vi "Partridge.vi"() -> ()   [LabVIEW 2012]
uses:
  <vilib>/picture/picture.llb/imagedata.ctl
  <vilib>/xml/Load XML String.vi
  <vilib>/xml/NI_XML.lvlib
  <resource>/objmgr/DOMUserDefRef.rc
panel:
  in  "XML Menu":string="<?xml version=\"1.0\" encoding=\"ISO-8859-1\"?>\n<Menu>\n<Starters>\n<Starter>\n<Name>Soup</Name>\n<Desc>A hearty winter vegetable soup.</Desc>\n</Starter>\n<Starter>\n<Name>Salmon</Name>\n<Desc>Scottish smoked salmon.</Desc>\n</Starter>\n</Starters>\n<Mains>\n<Main>\n<Name>Roast Turkey</Name>\n<Desc>With all the trimmings!</Desc>\n</Main>\n<Main>\n<Name>Fillet of Sea Bass</Name>\n<Desc>With lemon and thyme fondant.</Desc>\n</Main>\n<Main>\n<Name>Shepherd's Pie</Name>\n<Desc>With Puy lentils and vegetables.</Desc>\n</Main>\n</Mains>\n<Desserts>\n<Dessert>\n<Name>Christmas Pudding</Name>\n<Desc>The traditional favourite.</Desc>\n</Dessert>\n<Dessert>\n<Name>Rich Chocolate Tart</Name>\n<Desc>With orage chantilly creme.</Desc>\n</Dessert>\n</Desserts>\n</Menu>"
  in  "Christmas Tree View":string(tree)
  # "A Partridge in a Pear Tree"
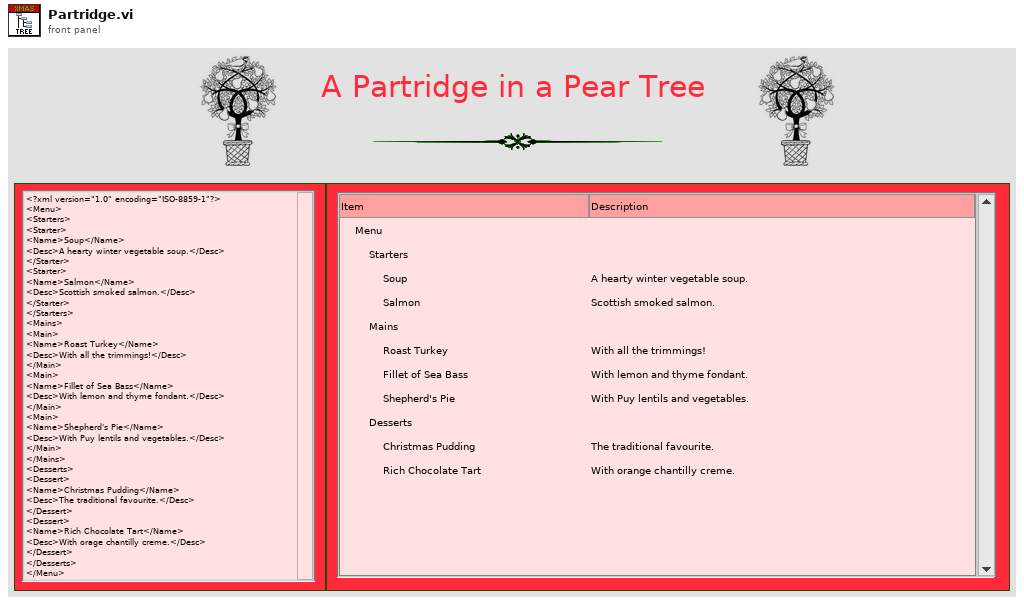
[diagram p1: front panel]
types:
  T1 = typedef "imagedata.ctl" = cluster{"image type":i32, "image depth":i32, "image":u8[], "mask":u8[], "colors":u32[], "Rectangle":cluster{"left":i16, "top":i16, "right":i16, "bottom":i16}}
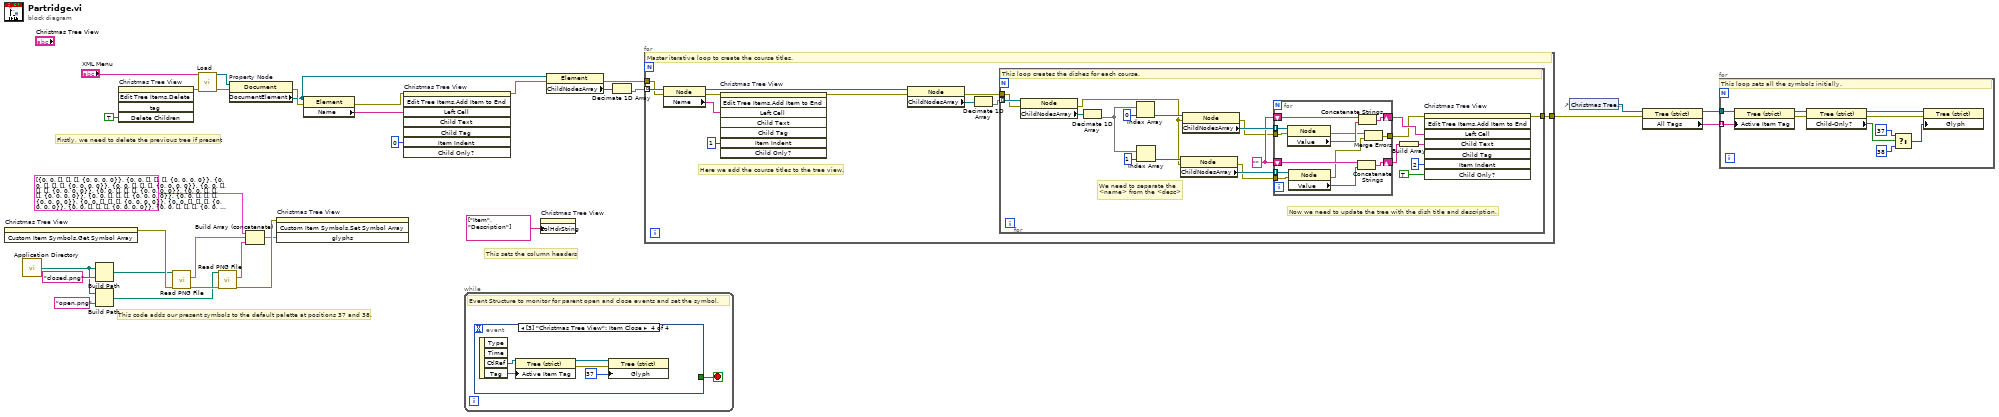
[diagram p0: block diagram]
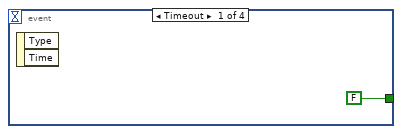
[diagram p2: hidden frame]
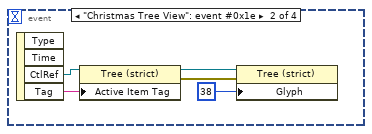
[diagram p3: hidden frame]
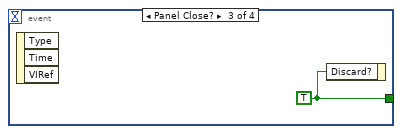
[diagram p4: hidden frame]
diagram:
  # "Firstly, we need to delete the previous tree if present"
  # "This sets the column headers"
  # "This code adds our present symbols to the default palette at positions 37 and 38."
  n1 = invoke on="Christmas Tree View" class="Tree (strict)" method="Custom Item Symbols.Get Symbol Array"() -> (error out=w19:errorcluster)  [unwired: 3 in, 2 out]
  n2 = call <vilib>:"Application Directory.vi"() -> ("Application Directory"=w14:path)
  n3 = Build Path(base path=w14, name or relative path="closed.png") -> (appended path=w13:path)
  n4 = Build Path(base path=w14, name or relative path="open.png") -> (appended path=w12:path)
  n5 = invoke on="Christmas Tree View" class="Tree (strict)" method="Edit Tree Items.Delete"("Delete Children"=TRUE ("Delete Children?")) -> (error out=w2:errorcluster)  [unwired: 4 in, 4 out]
  n6 = call <vilib>:"Read PNG File.vi"("error in (no error)"=w19, "path to PNG file"=w13) -> ("error out"=w18:errorcluster, "image data"=w11:T1)  [unwired: 7 in, 1 out]
  n7 = call-poly <vilib>:"Load.vi"("XML string"="XML Menu", "error in (no error)"=w2) -> ("DOM document out"=w31:refnum<k20>, "error out"=w30:errorcluster)  [unwired: 1 in, 11 out]
  n8 = call <vilib>:"Read PNG File.vi"("error in (no error)"=w18, "path to PNG file"=w12) -> ("error out"=w17:errorcluster, "image data"=w10:T1)  [unwired: 7 in, 1 out]
  n9 = property on="Property Node" class="Document"(reference=w31, error in=w30) -> (error out=w28:errorcluster, "DocumentElement"=w25:refnum<k20>)  [unwired: 1 out]
  n10 = Build Array (concatenate)(T1[] [{"image type"=0, "image depth"=0, "image"=[], "mask"=[], "colors"=[], "Rectangle"={"left"=0, "top"=0, "right"=0, "bottom"=0}}, {"image type"=0, "image depth"=0, "image"=[], "mask"=[], "colors"=[], "Rectangle"={"left"=0, "top"=0, "right"=0, "bottom"=0}}, {"image type"=0, "image depth"=0, "image"=[], "mask"=[], "colors"=[], "Rectangle"={"left"=0, "top"=0, "right"=0, "bottom"=0}}, {"image type"=0, "image depth"=0, "image"=[], "mask"=[], "colors"=[], "Rectangle"={"left"=0, "top"=0, "right"=0, "bottom"=0}}, {"image type"=0, "image depth"=0, "image"=[], "mask"=[], "colors"=[], "Rectangle"={"left"=0, "top"=0, "right"=0, "bottom"=0}}, {"image type"=0, "image depth"=0, "image"=[], "mask"=[], "colors"=[], "Rectangle"={"left"=0, "top"=0, "right"=0, "bottom"=0}}, {"image type"=0, "image depth"=0, "image"=[], "mask"=[], "colors"=[], "Rectangle"={"left"=0, "top"=0, "right"=0, "bottom"=0}}, {"image type"=0, "image depth"=0, "image"=[], "mask"=[], "colors"=[], "Rectangle"={"left"=0, "top"=0, "right"=0, "bottom"=0}}, {"image type"=0, "image depth"=0, "image"=[], "mask"=[], "colors"=[], "Rectangle"={"left"=0, "top"=0, "right"=0, "bottom"=0}}, {"image type"=0, "image depth"=0, "image"=[], "mask"=[], "colors"=[], "Rectangle"={"left"=0, "top"=0, "right"=0, "bottom"=0}}, {"image type"=0, "image depth"=0, "image"=[], "mask"=[], "colors"=[], "Rectangle"={"left"=0, "top"=0, "right"=0, "bottom"=0}}, {"image type"=0, "image depth"=0, "image"=[], "mask"=[], "colors"=[], "Rectangle"={"left"=0, "top"=0, "right"=0, "bottom"=0}}, {"image type"=0, "image depth"=0, "image"=[], "mask"=[], "colors"=[], "Rectangle"={"left"=0, "top"=0, "right"=0, "bottom"=0}}, {"image type"=0, "image depth"=0, "image"=[], "mask"=[], "colors"=[], "Rectangle"={"left"=0, "top"=0, "right"=0, "bottom"=0}}, {"image type"=0, "image depth"=0, "image"=[], "mask"=[], "colors"=[], "Rectangle"={"left"=0, "top"=0, "right"=0, "bottom"=0}}, {"image type"=0, "image depth"=0, "image"=[], "mask"=[], "colors"=[], "Rectangle"={"left"=0, "top"=0, "right"=0, "bottom"=0}}, {"image type"=0, "image depth"=0, "image"=[], "mask"=[], "colors"=[], "Rectangle"={"left"=0, "top"=0, "right"=0, "bottom"=0}}, {"image type"=0, "image depth"=0, "image"=[], "mask"=[], "colors"=[], "Rectangle"={"left"=0, "top"=0, "right"=0, "bottom"=0}}, {"image type"=0, "image depth"=0, "image"=[], "mask"=[], "colors"=[], "Rectangle"={"left"=0, "top"=0, "right"=0, "bottom"=0}}, {"image type"=0, "image depth"=0, "image"=[], "mask"=[], "colors"=[], "Rectangle"={"left"=0, "top"=0, "right"=0, "bottom"=0}}, {"image type"=0, "image depth"=0, "image"=[], "mask"=[], "colors"=[], "Rectangle"={"left"=0, "top"=0, "right"=0, "bottom"=0}}, {"image type"=0, "image depth"=0, "image"=[], "mask"=[], "colors"=[], "Rectangle"={"left"=0, "top"=0, "right"=0, "bottom"=0}}, {"image type"=0, "image depth"=0, "image"=[], "mask"=[], "colors"=[], "Rectangle"={"left"=0, "top"=0, "right"=0, "bottom"=0}}, {"image type"=0, "image depth"=0, "image"=[], "mask"=[], "colors"=[], "Rectangle"={"left"=0, "top"=0, "right"=0, "bottom"=0}}, {"image type"=0, "image depth"=0, "image"=[], "mask"=[], "colors"=[], "Rectangle"={"left"=0, "top"=0, "right"=0, "bottom"=0}}, {"image type"=0, "image depth"=0, "image"=[], "mask"=[], "colors"=[], "Rectangle"={"left"=0, "top"=0, "right"=0, "bottom"=0}}, {"image type"=0, "image depth"=0, "image"=[], "mask"=[], "colors"=[], "Rectangle"={"left"=0, "top"=0, "right"=0, "bottom"=0}}, {"image type"=0, "image depth"=0, "image"=[], "mask"=[], "colors"=[], "Rectangle"={"left"=0, "top"=0, "right"=0, "bottom"=0}}, {"image type"=0, "image depth"=0, "image"=[], "mask"=[], "colors"=[], "Rectangle"={"left"=0, "top"=0, "right"=0, "bottom"=0}}, {"image type"=0, "image depth"=0, "image"=[], "mask"=[], "colors"=[], "Rectangle"={"left"=0, "top"=0, "right"=0, "bottom"=0}}, {"image type"=0, "image depth"=0, "image"=[], "mask"=[], "colors"=[], "Rectangle"={"left"=0, "top"=0, "right"=0, "bottom"=0}}, {"image type"=0, "image depth"=0, "image"=[], "mask"=[], "colors"=[], "Rectangle"={"left"=0, "top"=0, "right"=0, "bottom"=0}}, {"image type"=0, "image depth"=0, "image"=[], "mask"=[], "colors"=[], "Rectangle"={"left"=0, "top"=0, "right"=0, "bottom"=0}}, {"image type"=0, "image depth"=0, "image"=[], "mask"=[], "colors"=[], "Rectangle"={"left"=0, "top"=0, "right"=0, "bottom"=0}}, {"image type"=0, "image depth"=0, "image"=[], "mask"=[], "colors"=[], "Rectangle"={"left"=0, "top"=0, "right"=0, "bottom"=0}}, {"image type"=0, "image depth"=0, "image"=[], "mask"=[], "colors"=[], "Rectangle"={"left"=0, "top"=0, "right"=0, "bottom"=0}}, {"image type"=0, "image depth"=0, "image"=[], "mask"=[], "colors"=[], "Rectangle"={"left"=0, "top"=0, "right"=0, "bottom"=0}}], w11, w10) -> (w9:T1[])
  n11 = invoke on="Christmas Tree View" class="Tree (strict)" method="Custom Item Symbols.Set Symbol Array"(error in=w17, "glyphs"=w9) -> ()  [unwired: 2 in, 4 out]
  n12 = property class="Element"(reference=w25, error in=w28) -> (error out=w27:errorcluster, "Name"=w7:string)  [unwired: 1 out]
  n13 = invoke on="Christmas Tree View" class="Tree (strict)" method="Edit Tree Items.Add Item to End"(error in=w27, "Left Cell"=w7, "Item Indent"=0 ("New Item Indentation")) -> (error out=w24:errorcluster)  [unwired: 5 in, 7 out]
  n14 = while {
    stop <- w32 stop-if-true
    # "Event Structure to monitor for parent open and close events and set the symbol."
    n15 = event shown="[3] \"Christmas Tree View\": Item Close" {
      selector: _ -> [_ _ _ _]
      dyn-events: _ -> [_ _ _ _]
      timeout: _ -> [_ _ _ _]
      tunnel: [FALSE ("Stop Button") _ w39 _] -> w32
      event Timeout {
        n16 = event-data() -> ()  [unwired: 1 in, 2 out]
      }
      event "Christmas Tree View": event #0x1e {
        n17 = event-data() -> ("CtlRef"=w34:refnum<vi>, "Tag"=w38:string)  [unwired: 1 in, 2 out]
        n18 = property class="Tree (strict)"(reference=w34, "Active Item Tag"=w38) -> (reference out=w35:refnum<vi>, error out=w36:errorcluster)  [unwired: 1 in]
        n19 = property class="Tree (strict)"(reference=w35, error in=w36, "Glyph"=38 ("Active Item:Symbol Index")) -> ()  [unwired: 2 out]
      }
      event Panel Close? {
        w39 = TRUE ("Stop Button")
        n20 = event-data() -> ()  [unwired: 1 in, 3 out]
        n21 = event-data("Discard?"=w39) -> ()  [unwired: 1 in, 1 out]
      }
      event "Christmas Tree View": Item Close {
        n22 = event-data() -> ("CtlRef"=w40:refnum<vi>, "Tag"=w41:string)  [unwired: 1 in, 2 out]
        n23 = property class="Tree (strict)"(reference=w40, "Active Item Tag"=w41) -> (reference out=w44:refnum<vi>, error out=w43:errorcluster)  [unwired: 1 in]
        n24 = property class="Tree (strict)"(reference=w44, error in=w43, "Glyph"=37 ("Active Item:Symbol Index")) -> ()  [unwired: 2 out]
      }
    }
  }
  n25 = property on="Christmas Tree View" class="Tree (strict)"("ColHdrString"=string[] ["Item", "Description"]) -> ()  [unwired: 2 in, 2 out]
  n26 = property class="Element"(reference=w25, error in=w24) -> (error out=w22:errorcluster, "ChildNodesArray"=w23:refnum<k20>[])  [unwired: 1 out]
  n27 = Decimate 1D Array(w23) -> (w21:refnum<k20>[])  [unwired: 1 out]
  n28 = for {
    tunnel: w21 -> [w55] mode=indexing
    tunnel: w22 -> [w47]
    tunnel: [w45] -> w4
    # "Here we add the course titles to the tree view."
    # "Master iterative loop to create the course titles."
    n29 = property class="Node"(reference=w55, error in=w47) -> (reference out=w51:refnum<k20>, error out=w54:errorcluster, "Name"=w53:string)
    n30 = invoke on="Christmas Tree View" class="Tree (strict)" method="Edit Tree Items.Add Item to End"(error in=w54, "Left Cell"=w53, "Item Indent"=1 ("New Item Indentation")) -> (error out=w50:errorcluster)  [unwired: 5 in, 7 out]
    n31 = property class="Node"(reference=w51, error in=w50) -> (error out=w46:errorcluster, "ChildNodesArray"=w49:refnum<k20>[])  [unwired: 1 out]
    n32 = Decimate 1D Array(w49) -> (w48:refnum<k20>[])  [unwired: 1 out]
    n33 = for {
      tunnel: w48 -> [w76] mode=indexing
      tunnel: w46 -> [w61]
      tunnel: [w56] -> w45
      w67 = ""
      # "Now we need to update the tree with the dish title and description."
      # "We need to separate the\n<name> from the <desc>"
      # "This loop creates the dishes for each course."
      n34 = property class="Node"(reference=w76, error in=w61) -> (error out=w58:errorcluster, "ChildNodesArray"=w75:refnum<k20>[])  [unwired: 1 out]
      n35 = Decimate 1D Array(w75) -> (w72:refnum<k20>[])  [unwired: 1 out]
      n36 = Index Array(array=w72, index=0) -> (element=w73:refnum<k20>)
      n37 = Index Array(array=w72, index=1) -> (element=w69:refnum<k20>)
      n38 = property class="Node"(reference=w69, error in=w58) -> (error out=w59:errorcluster, "ChildNodesArray"=w68:refnum<k20>[])  [unwired: 1 out]
      n39 = property class="Node"(reference=w73, error in=w58) -> (error out=w60:errorcluster, "ChildNodesArray"=w74:refnum<k20>[])  [unwired: 1 out]
      n40 = for {
        tunnel: w74 -> [w82] mode=indexing
        shift-right: [w88] -> w65
        shift-left: w67 -> [w89]
        shift-right: [w87] -> w66
        shift-left: w67 -> [w86]
        tunnel: w68 -> [w83] mode=indexing
        tunnel: w60 -> [w81]
        tunnel: w59 -> [w80]
        tunnel: [w77] -> w57
        n41 = property class="Node"(reference=w82, error in=w81) -> (error out=w79:errorcluster, "Value"=w85:string)  [unwired: 1 out]
        n42 = property class="Node"(reference=w83, error in=w80) -> (error out=w78:errorcluster, "Value"=w84:string)  [unwired: 1 out]
        n43 = Concatenate Strings(w89, w84) -> (w88:string)
        n44 = Concatenate Strings(w86, w85) -> (w87:string)
        n45 = Merge Errors(w79, w78) -> (w77:errorcluster)
      }
      n46 = Build Array(w65) -> (w64:string[])
      n47 = invoke on="Christmas Tree View" class="Tree (strict)" method="Edit Tree Items.Add Item to End"(error in=w57, "Left Cell"=w66, "Child Text"=w64, "Item Indent"=2 ("New Item Indentation"), "Child Only?"=TRUE) -> (error out=w56:errorcluster)  [unwired: 3 in, 7 out]
    }
  }
  n48 = control-ref of="Christmas Tree View"() -> (w3:refnum<vi>)
  n49 = property class="Tree (strict)"(reference=w3, error in=w4) -> (reference out=w5:refnum<vi>, "All Tags"=w6:string[])  [unwired: 1 out]
  n50 = for {
    tunnel: w6 -> [w99] mode=indexing
    tunnel: w5 -> [w98]
    # "This loop sets all the symbols initially."
    n51 = property class="Tree (strict)"(reference=w98, "Active Item Tag"=w99) -> (reference out=w97:refnum<vi>, error out=w96:errorcluster)  [unwired: 1 in]
    n52 = property class="Tree (strict)"(reference=w97, error in=w96) -> (reference out=w91:refnum<vi>, error out=w90:errorcluster, "Child-Only?"=w93:bool)
    n53 = Select(t=37 ("Active Item:Symbol Index"), s=w93, f=38 ("Active Item:Symbol Index")) -> (s? t:f=w92:i32)
    n54 = property class="Tree (strict)"(reference=w91, error in=w90, "Glyph"=w92) -> ()  [unwired: 2 out]
  }
